vi "Task Type.vi"(11 "DebugGUI in":refnum<class "DebugGUI.lvclass">) -> (2 "Task Type":string)   [LabVIEW 2020, in "Volatus.lvlib" / "DebugGUI.lvclass"]
uses:
  DebugGUI.lvclass
  DebugGUI.lvclass/DebugGUI.ctl
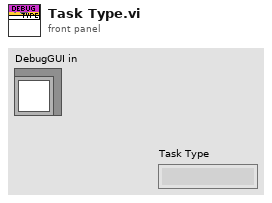
[diagram p1: front panel]
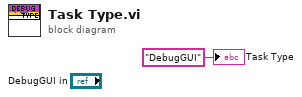
[diagram p0: block diagram]
diagram:
  "Task Type" <- "DebugGUI" ("Task Type")
